vi "ToArray.vi"(8 "error in":errorcluster, 11 "Generic in":refnum<class "Generic.lvclass">) -> (0 "error out":errorcluster, 3 "Array out":refnum<class "Array.lvclass">)   [LabVIEW 2014, in "Array.lvclass"]
uses:
  Array.lvclass
  Generic/Generic.lvclass
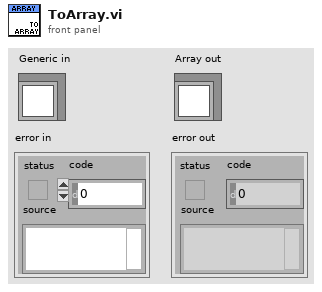
[diagram p1: front panel]
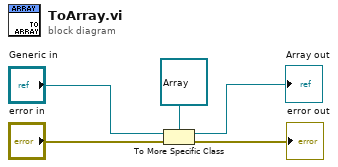
[diagram p0: block diagram]
diagram:
  n1 = To More Specific Class(target class=refnum<class "Array.lvclass"> refnum ("Array in"), reference="Generic in", error in="error in") -> (specific class reference=→"Array out":refnum<class "Array.lvclass">, error out=→"error out":errorcluster)
